vi "Volt Channels.vi"(11 "Sensor List Class in":refnum<class "Sensor List Class.lvclass">) -> (2 "Volt Channels":string[](array[string]), 3 "Sensor List Class out":refnum<class "Sensor List Class.lvclass">)   [LabVIEW 2013]
uses:
  Data Access Objects/Sensors/Sensor List Class.lvclass
  Data Access Objects/Sensors/Sensor DAO Class.lvclass/Sensor DAO Class.ctl
  <vilib>/regexp/Match Regular Expression.xnode
  Data Access Objects/Sensors/Sensor DAO Class.lvclass
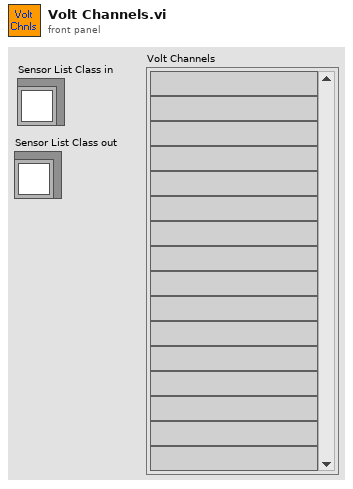
[diagram p1: front panel]
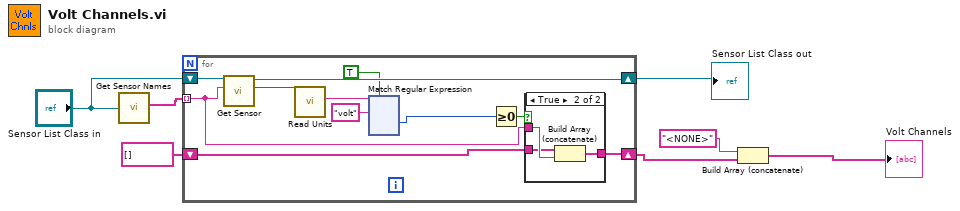
[diagram p0: block diagram]
diagram:
  n1 = call "Get Sensor Names.vi"("Sensor List Class in"="Sensor List Class in") -> ("Names"=w5:string[])  [unwired: 8 in, 2 out]
  n2 = for {
    shift-right: [w18] -> w6
    shift-left: string[] [] -> [w17]
    tunnel: w5 -> [w8] mode=indexing
    shift-right: [w15] -> w7
    shift-left: "Sensor List Class in" -> [w16]
    n3 = call "Get Sensor.vi"("Name"=w8, "Sensor List Class in"=w16) -> ("Sensor DAO Out"=w14:refnum<class "Sensor DAO Class.lvclass">, "Sensor List Class out"=w15:refnum<class "Sensor List Class.lvclass">)  [unwired: 7 in, 1 out]
    n4 = call "Read Units.vi"("Sensor DAO Class in"=w14) -> ("Units"=w13:string)  [unwired: 8 in, 2 out]
    n5 = xnode "Match Regular Expression"("input string"=w13, "regular expression"="volt", "ignore case? (F)"=TRUE) -> ("offset past match"=w11:i32)  [unwired: 3 in, 4 out]
    n6 = Greater Or Equal To 0?(x=w11) -> (x >= 0?=w12:bool)
    n7 = case shown="True" w12 {
      tunnel: w8 -> [_ w136]
      tunnel: [w133 w135] -> w18
      tunnel: w17 -> [w133 w134]
      frame False {
      }
      frame True {
        n8 = Build Array (concatenate)(w134, w136) -> (w135:string[])
      }
    }
  }
  "Sensor List Class out" <- w7
  n9 = Build Array (concatenate)("<NONE>", w6) -> (→"Volt Channels":string[])
